vi "filter focus.vi"(11 "Z focus":cluster{dbl[], "histogram plot":dbl[]}(graph)={[4.449999999999826, 4.454999999999826, 4.459999999999826, 4.464999999999826, 4.469999999999826, 4.474999999999826, 4.4799999999998255, 4.484999999999825, 4.489999999999825, 4.494999999999825, 4.499999999999825, 4.504999999999825, 4.509999999999825, 4.514999999999825, 4.519999999999825, 4.5249999999998245, 4.529999999999824, 4.534999999999824, 4.539999999999824, 4.544999999999824, 4.549999999999824, 4.554999999999824, 4.559999999999824, 4.564999999999824, 4.5699999999998235, 4.574999999999823, 4.579999999999823, 4.584999999999823, 4.589999999999823, 4.594999999999823, 4.599999999999823, 4.604999999999823, 4.609999999999823, 4.614999999999823, 4.6199999999998225, 4.624999999999822, 4.629999999999822, 4.634999999999822, 4.639999999999822, 4.644999999999822, 4.649999999999822], "histogram plot"=[7860.0, 9920.0, 8180.0, 9320.0, 10900.0, 10880.0, 10400.0, 11020.0, 12200.0, 11300.0, 10740.0, 11160.0, 10860.0, 11860.0, 10080.0, 11520.0, 9920.0, 10680.0, 9840.0, 9600.0, 9460.0, 9540.0, 10180.0, 9600.0, 8560.0, 10440.0, 9220.0, 9300.0, 9600.0, 9360.0, 9280.0, 8940.0, 8620.0, 8420.0, 7860.0, 7960.0, 7160.0, 8440.0, 7780.0, 7800.0, 6660.0]}) -> (3 "filtered focus":cluster{dbl[], "histogram plot":dbl[]}(graph)={[4.449999999999826, 4.454999999999826, 4.459999999999826, 4.464999999999826, 4.469999999999826, 4.474999999999826, 4.4799999999998255, 4.484999999999825, 4.489999999999825, 4.494999999999825, 4.499999999999825, 4.504999999999825, 4.509999999999825, 4.514999999999825, 4.519999999999825, 4.5249999999998245, 4.529999999999824, 4.534999999999824, 4.539999999999824, 4.544999999999824, 4.549999999999824, 4.554999999999824, 4.559999999999824, 4.564999999999824, 4.5699999999998235, 4.574999999999823, 4.579999999999823, 4.584999999999823, 4.589999999999823, 4.594999999999823, 4.599999999999823, 4.604999999999823, 4.609999999999823, 4.614999999999823, 4.6199999999998225, 4.624999999999822, 4.629999999999822, 4.634999999999822, 4.639999999999822, 4.644999999999822, 4.649999999999822], "histogram plot"=[7860.0, 9920.0, 8180.0, 9320.0, 10900.0, 10880.0, 10400.0, 11020.0, 12200.0, 11300.0, 10740.0, 11160.0, 10860.0, 11860.0, 10080.0, 11520.0, 9920.0, 10680.0, 9840.0, 9600.0, 9460.0, 9540.0, 10180.0, 9600.0, 8560.0, 10440.0, 9220.0, 9300.0, 9600.0, 9360.0, 9280.0, 8940.0, 8620.0, 8420.0, 7860.0, 7960.0, 7160.0, 8440.0, 7780.0, 7800.0, 6660.0]})   [LabVIEW 2014]
uses:
  <vilib>/Analysis/NI_AALBase.lvlib
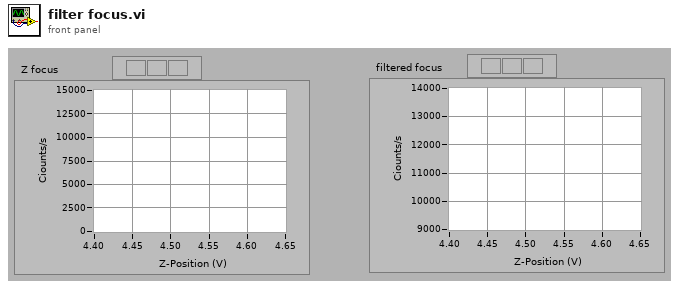
[diagram p1: front panel]
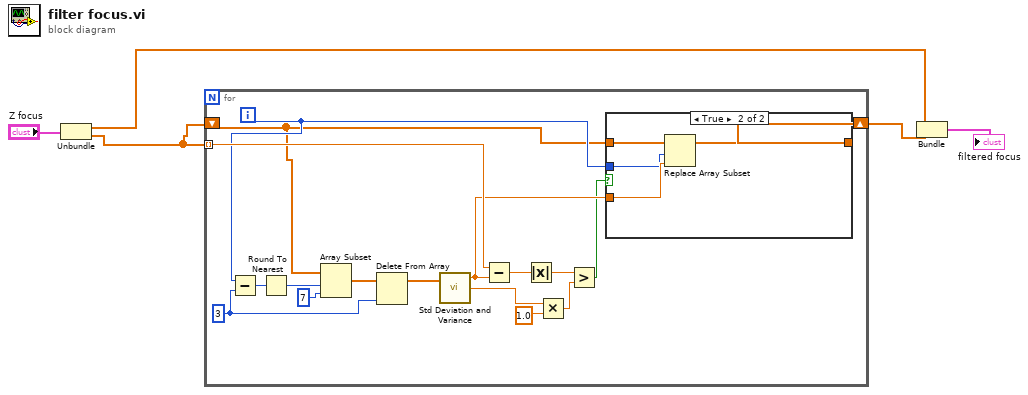
[diagram p0: block diagram]
diagram:
  n1 = Unbundle("Z focus") -> (w2:dbl[], "histogram plot"=w1:dbl[])
  n2 = for {
    tunnel: w1 -> [w21] mode=indexing
    shift-right: [w16] -> w4
    shift-left: w1 -> [w7]
    i -> [w13]
    w10 = 3 ("y")
    n3 = Subtract(x=w13, y=w10) -> (x-y=w22:i32)
    n4 = Round To Nearest(number=w22) -> (nearest integer value=w15:i32)
    n5 = Array Subset(array=w7, index=w15, length=7) -> (w14:dbl[])
    n6 = Delete From Array(array=w14, index=w10) -> (array with subset deleted=w12:dbl[])  [unwired: 1 in, 1 out]
    n7 = call <vilib>:"Std Deviation and Variance.vi"("X"=w12) -> ("mean"=w8:dbl, "standard deviation"=w19:dbl)  [unwired: 1 in, 1 out]
    n8 = Subtract(x=w21, y=w8) -> (x-y=w20:dbl)
    n9 = Absolute Value(x=w20) -> (abs(x)=w9:dbl)
    n10 = Multiply(x=w19, y=1.0) -> (x*y=w17:dbl)
    n11 = Greater?(x=w9, y=w17) -> (0:w6:bool)
    n12 = case shown="True" w6 {
      tunnel: [w23 w25] -> w16
      tunnel: w7 -> [w23 w27]
      tunnel: w13 -> [_ w24]
      tunnel: w8 -> [_ w26]
      frame False {
      }
      frame True {
        n13 = Replace Array Subset(array=w27, new element=w26, index=w24) -> (w25:dbl[])
      }
    }
  }
  n14 = Bundle(w2, "histogram plot"=w4) -> (→"filtered focus":cluster{dbl[], "histogram plot":dbl[]})  [unwired: 1 in]
